vi "Repos_Handler.vi"(8 "Error In":errorcluster caption="Entrée d'erreur", 11 "Donnees_Globales_IN":T1) -> (0 "Error Out":errorcluster, 3 "Donnees_Globale_Out":T1)   [LabVIEW 2019]
uses:
  Asc_State_Inputs.ctl
  Etat_Asc.ctl
  <vilib>/Utility/error.llb/Error Cluster From Error Code.vi
  <vilib>/rvi/errors/niLvFpgaAdjustHostInterfaceError.vi
  <vilib>/rvi/interface/nirviReadWriteControl/nirviReadWriteControl.xnode
  NiFpgaLv.dll
  <vilib>/rvi/interface/Simulation/niFpgaSimulationCallBeginRW.vi
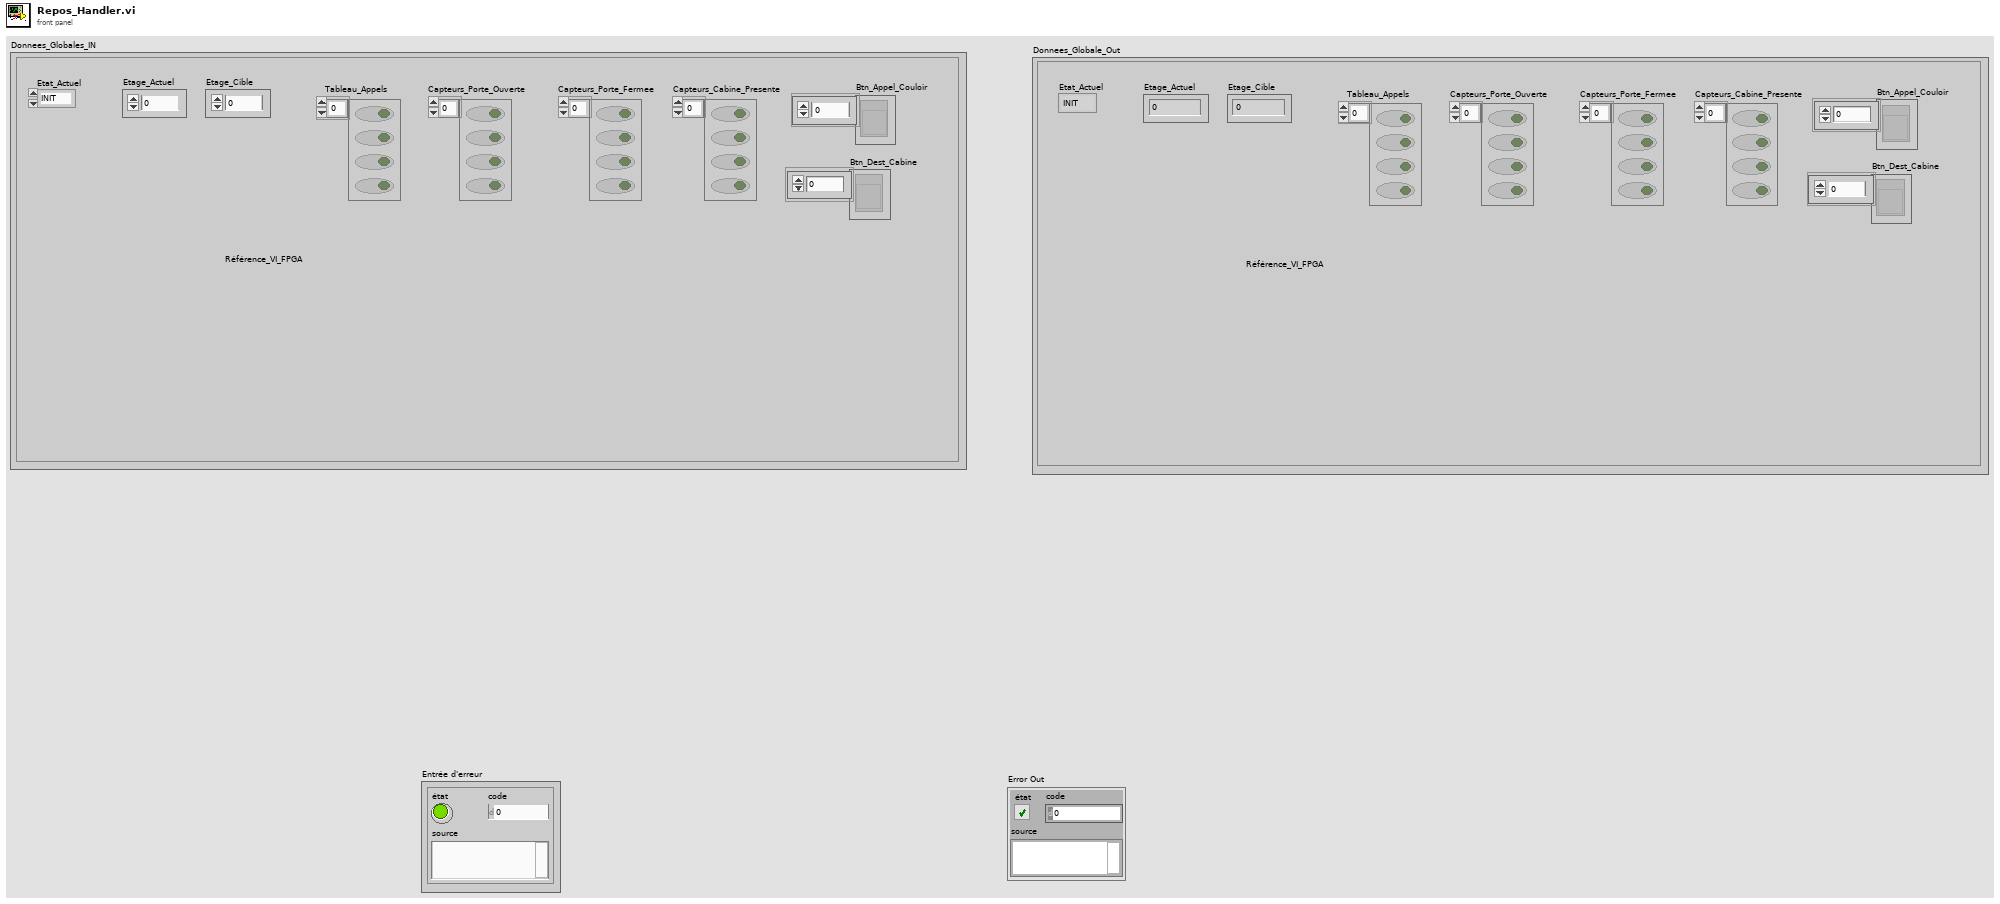
[diagram p1: front panel]
types:
  T1 = typedef "Asc_State_Inputs.ctl" = cluster{"Etage_Actuel":i32, "Etat_Actuel":T2, "Etage_Cible":i32, "Tableau_Appels":bool[], "Capteurs_Porte_Ouverte":bool[], "Capteurs_Porte_Fermee":bool[], "Capteurs_Cabine_Presente":bool[], "Btn_Appel_Couloir":refnum<vi>[], "Btn_Dest_Cabine":refnum<vi>[], "Référence_VI_FPGA":refnum<k20>}
  T2 = typedef "Etat_Asc.ctl" = enum16{"INIT", "REPOS", "DEPLACEMENT", "OUVERTURE_PORTE", "ATTENTE_TEMPO", "FERMETURE_PORTE", "ARRET_URGENCE"}
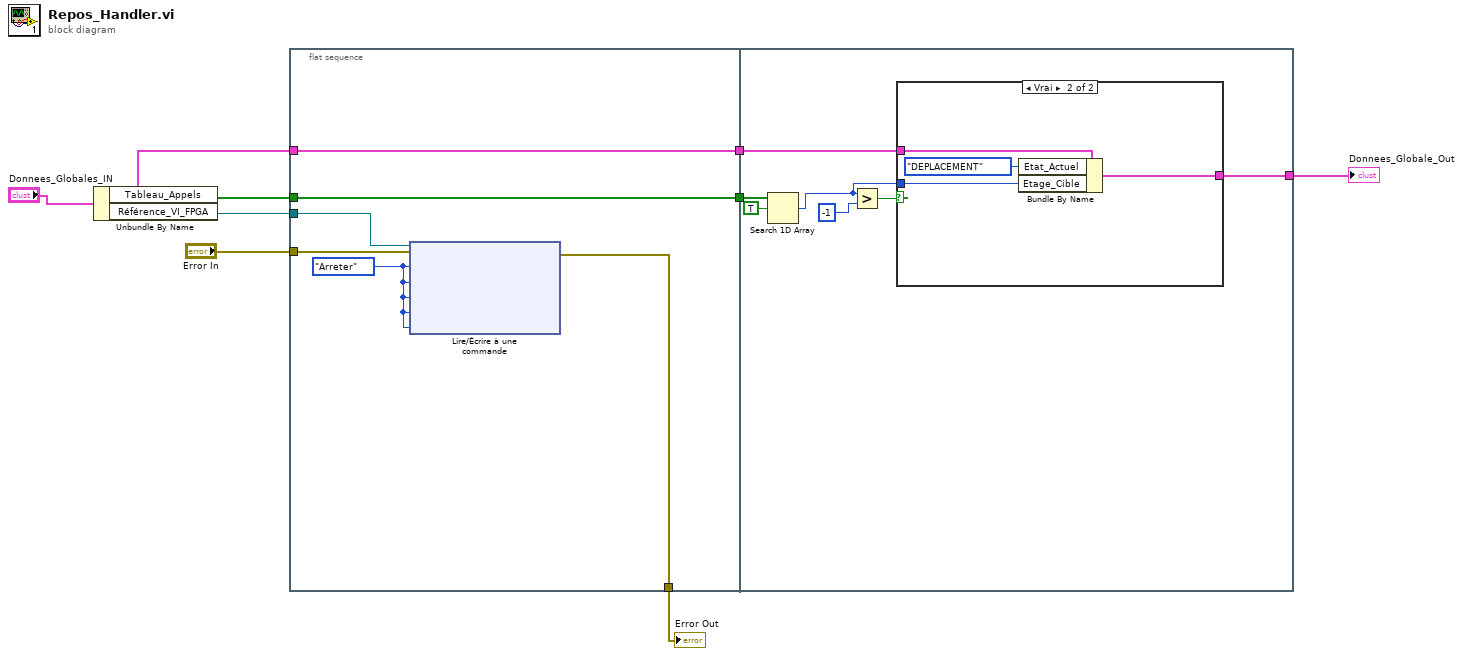
[diagram p0: block diagram]
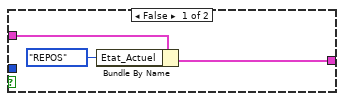
[diagram p2: hidden frame]
diagram:
  n1 = Unbundle By Name("Donnees_Globales_IN") -> ("Tableau_Appels"=w8:bool[], "Référence_VI_FPGA"=w3:refnum<k20>)
  n2 = flat-sequence {
    tunnel: "Donnees_Globales_IN" -> [w13]
    tunnel: w8 -> [w14]
    tunnel: [w14] -> w5
    tunnel: [w13] -> w4
    tunnel: w3 -> [w12]
    tunnel: "Error In" -> [w10]
    tunnel: [w9] -> w1
    tunnel: [w15] -> w6
    tunnel: w5 -> [w21]
    tunnel: w4 -> [w17]
    frame #0 {
      w11 = enum16{"Monter", "Descendre", "Arreter"}."Arreter" ("CMD_Moteur_Cabine")
      n3 = xnode "Lire/Écrire à une commande"("Référence de VI FPGA en entrée"=w12, "entrée d'erreur"=w10, "CMD_Moteur_Cabine"=w11, "CMD_Moteur_Porte_RDC"=w11, "CMD_Moteur_Porte_1"=w11, "CMD_Moteur_Porte_2"=w11, "CMD_Moteur_Porte_3"=w11) -> ("sortie d'erreur"=w9:errorcluster)  [unwired: 1 out]
    }
    frame #1 {
      n4 = Search 1D Array(1D array=w21, element=TRUE ("élément")) -> (index of element=w16:i32)  [unwired: 1 in]
      n5 = Greater?(x=w16, y=-1) -> (0:w18:bool)
      n6 = case shown="Vrai" w18 {
        tunnel: w17 -> [w24 w28]
        tunnel: w16 -> [_ w26]
        tunnel: [w22 w25] -> w15
        frame False {
          n7 = Bundle By Name(cluster=w24, "Etat_Actuel"=Etat_Asc."REPOS") -> (w22:T1)
        }
        frame True {
          n8 = Bundle By Name(cluster=w28, "Etat_Actuel"=Etat_Asc."DEPLACEMENT", "Etage_Cible"=w26) -> (w25:T1)
        }
      }
    }
  }
  "Donnees_Globale_Out" <- w6
  "Error Out" <- w1
